vi "Update Wall State.vi"(10 "wall state in":T1, 11 "map in":refnum<data-value>) -> (2 "wall state out":T1, 3 "map out":refnum<data-value>)   [LabVIEW 2020, in "Great Wall.lvclass"]
uses:
  Great Wall.lvclass
  DS Square Library/Mapping/Map.ctl
  DS Square Library/Mapping/Square Status.ctl
  DS Square Library/Mapping/Square State.ctl
  DS Square Library/Mapping/Center of Mass.ctl
  Wall State.ctl
  Wall State Enum.ctl
  Type Defs/Direction Enum.ctl
  Common/Position.ctl
  SubVIs/Read-Only Globals.vi
  SubVIs/Globals (private).vi
  DS Square Library/DS Square.lvlib
  Common/Common.lvlib
  Square/Square.lvclass
  Type Defs/SB Type Defs.lvlib
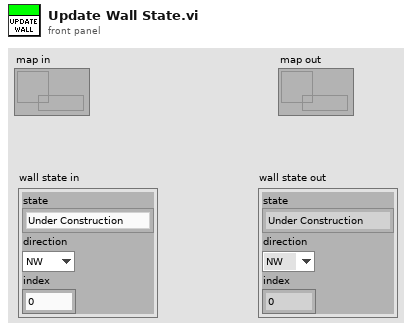
[diagram p1: front panel]
types:
  T1 = typedef "Great Wall.lvclass/Wall State.ctl" = cluster{"state":T2, "direction":T3, "index":i32}
  T2 = typedef "Great Wall.lvclass/Wall State Enum.ctl" = enum16{"Under Construction", "Hold", "Advance 1", "Advance 2", "Retreat"}
  T3 = typedef "SB Type Defs.lvlib/Direction Enum.ctl" = enum16{"NW", "N", "NE", "E", "SE", "S", "SW", "W"}
  T4 = typedef "DS Square.lvlib/Square State.ctl" = enum16{"Unknown", "Empty", "Occupied - Active", "Occupied - Cool Down", "Attacked", "Enemy", "Enemy Wall"}
  T5 = typedef "Common.lvlib/Position.ctl" = cluster{"Column":i32, "Row":i32}
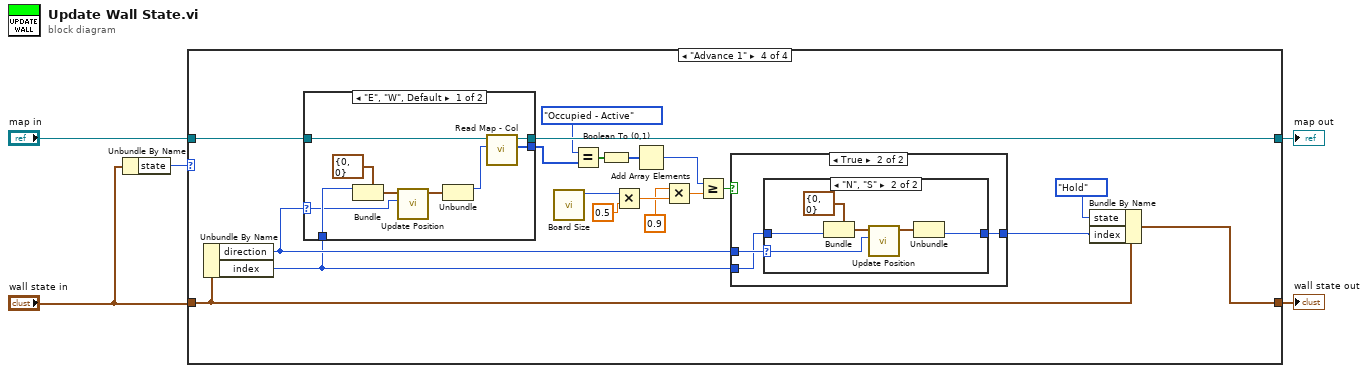
[diagram p0: block diagram]
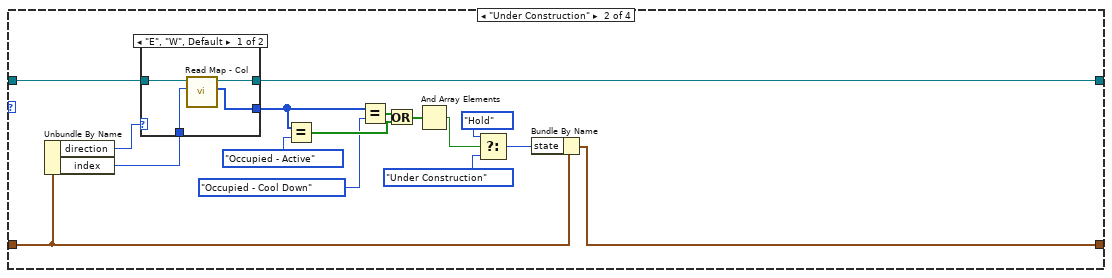
[diagram p3: hidden frame]
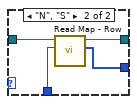
[diagram p4: hidden frame]
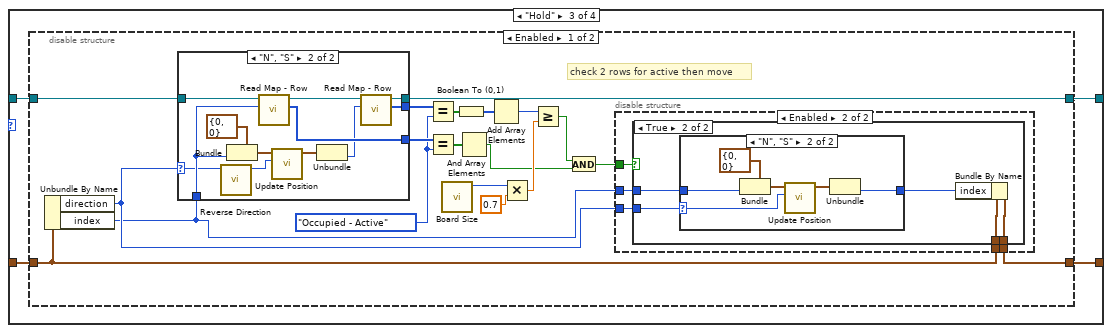
[diagram p5: hidden frame]
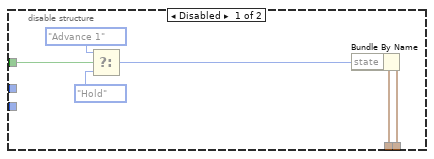
[diagram p6: hidden frame]
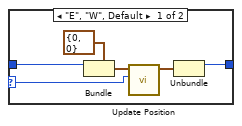
[diagram p8: hidden frame]
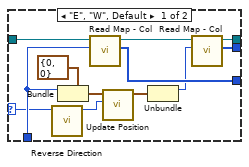
[diagram p9: hidden frame]
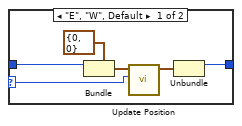
[diagram p12: hidden frame]
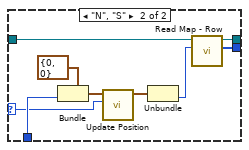
[diagram p13: hidden frame]
diagram:
  n1 = Unbundle By Name("wall state in") -> ("state"=w3:T2)
  n2 = case shown="\"Advance 1\"" w3 {
    tunnel: "map in" -> [w7 w17 w35 w127]
    tunnel: [w7 w16 w34 w126] -> w4
    tunnel: "wall state in" -> [w6 w13 w33 w125]
    tunnel: [w6 w8 w32 w128] -> w1
    frame Default {
    }
    frame "Under Construction" {
      n3 = Unbundle By Name(w13) -> ("direction"=w15:T3, "index"=w14:i32)
      n4 = case shown="\"E\", \"W\", Default" w15 {
        tunnel: w17 -> [w27 w31]
        tunnel: w14 -> [w24 w30]
        tunnel: [w26 w29] -> w16
        tunnel: [w25 w28] -> w19
        frame "E", "W", Default {
          n5 = call "Read Map - Col.vi"("Column"=w24, "map in"=w27) -> ("square states"=w25:T4[], "map out"=w26:refnum<data-value>)  [unwired: 8 in]
        }
        frame "N", "S" {
          n6 = call "Read Map - Row.vi"("Row"=w30, "map"=w31) -> ("square states"=w28:T4[], "map"=w29:refnum<data-value>)  [unwired: 8 in]
        }
      }
      n7 = Equal?(x=w19, y=Square_State."Occupied - Active" ("square state")) -> (x = y?=w22:bool[])
      n8 = Equal?(x=w19, y=Square_State."Occupied - Cool Down" ("square state")) -> (x = y?=w21:bool[])
      n9 = Or(x=w21, y=w22) -> (x .or. y?=w23:bool[])
      n10 = And Array Elements(Boolean array=w23) -> (logical AND=w12:bool)
      n11 = Select(t=Wall_State_Enum."Hold" ("state"), s=w12, f=Wall_State_Enum."Under Construction" ("state")) -> (s? t:f=w9:T2)
      n12 = Bundle By Name(cluster=w13, "state"=w9) -> (w8:T1)
    }
    frame "Hold" {
      n13 = disable-structure shown="Enabled" {
        disable-tunnel: w35 -> [w53 w109]
        disable-tunnel: [w52 w109] -> w34
        disable-tunnel: w33 -> [w51 w108]
        disable-tunnel: [w50 w108] -> w32
        frame Enabled {
          w47 = Square_State."Occupied - Active" ("square state")
          # "check 2 rows for active then move"
          n14 = Unbundle By Name(w51) -> ("direction"=w37:T3, "index"=w36:i32)
          n15 = case shown="\"N\", \"S\"" w37 {
            selector: w37 -> [w85 w97]
            tunnel: w53 -> [w95 w107]
            tunnel: w36 -> [w87 w99]
            tunnel: [w90 w102] -> w52
            tunnel: [w89 w101] -> w54
            tunnel: [w88 w100] -> w48
            frame "E", "W", Default {
              n16 = call "Reverse Direction.vi"("Direction in"=w85) -> ("Reverse Direction"=w84:i32)  [unwired: 10 in]
              n17 = Bundle(cluster=T5 {"Column"=0, "Row"=0} ("Position in"), "Column"=w87) -> (w93:T5)  [unwired: 1 in]
              n18 = call "Read Map - Col.vi"("Column"=w87, "map in"=w95) -> ("square states"=w89:T4[], "map out"=w91:refnum<data-value>)  [unwired: 8 in]
              n19 = call "Update Position.vi"("Direction"=w84, "Position in"=w93) -> ("Position out"=w92:T5)  [unwired: 9 in]
              n20 = Unbundle(w92) -> ("Column"=w86:i32)  [unwired: 1 out]
              n21 = call "Read Map - Col.vi"("Column"=w86, "map in"=w91) -> ("square states"=w88:T4[], "map out"=w90:refnum<data-value>)  [unwired: 8 in]
            }
            frame "N", "S" {
              n22 = call "Reverse Direction.vi"("Direction in"=w97) -> ("Reverse Direction"=w96:i32)  [unwired: 10 in]
              n23 = Bundle(cluster=T5 {"Column"=0, "Row"=0} ("Position in"), "Row"=w99) -> (w105:T5)  [unwired: 1 in]
              n24 = call "Read Map - Row.vi"("Row"=w99, "map"=w107) -> ("square states"=w101:T4[], "map"=w103:refnum<data-value>)  [unwired: 8 in]
              n25 = call "Update Position.vi"("Direction"=w96, "Position in"=w105) -> ("Position out"=w104:T5)  [unwired: 9 in]
              n26 = Unbundle(w104) -> ("Row"=w98:i32)  [unwired: 1 out]
              n27 = call "Read Map - Row.vi"("Row"=w98, "map"=w103) -> ("square states"=w100:T4[], "map"=w102:refnum<data-value>)  [unwired: 8 in]
            }
          }
          n28 = Equal?(x=w48, y=w47) -> (x = y?=w46:bool[])
          n29 = Equal?(x=w54, y=w47) -> (x = y?=w49:bool[])
          n30 = call "Board Size.vi"() -> ("Board Size"=w44:i32)  [unwired: 11 in]
          n31 = Boolean To (0,1)(Boolean=w46) -> (0, 1=w45:i16[])
          n32 = And Array Elements(Boolean array=w49) -> (logical AND=w39:bool)
          n33 = Add Array Elements(numeric array=w45) -> (sum=w42:i16)
          n34 = Multiply(x=w44, y=0.7) -> (x*y=w41:dbl)
          n35 = Greater Or Equal?(x=w42, y=w41) -> (x >= y?=w40:bool)
          n36 = And(x=w40, y=w39) -> (x .and. y?=w38:bool)
          n37 = disable-structure shown="Enabled" {
            disable-tunnel: w51 -> [w60 w61]
            disable-tunnel: [w56 w62] -> w50
            disable-tunnel: w38 -> [w55 w64]
            disable-tunnel: w37 -> [_ w65]
            disable-tunnel: w36 -> [_ w63]
            frame Disabled {
              n38 = Select(t=Wall_State_Enum."Advance 1" ("state"), s=w55, f=Wall_State_Enum."Hold" ("state")) -> (s? t:f=w57:T2)
              n39 = Bundle By Name(cluster=w60, "state"=w57) -> (w56:T1)
            }
            frame Enabled {
              n40 = case shown="True" w64 {
                tunnel: w65 -> [_ w71]
                tunnel: w63 -> [_ w70]
                tunnel: [w66 w69] -> w62
                tunnel: w61 -> [w66 w68]
                frame False {
                }
                frame True {
                  n41 = case shown="\"N\", \"S\"" w71 {
                    selector: w71 -> [w72 w78]
                    tunnel: w70 -> [w74 w80]
                    tunnel: [w73 w79] -> w67
                    frame "E", "W", Default {
                      n42 = Bundle(cluster=T5 {"Column"=0, "Row"=0} ("Position in"), "Column"=w74) -> (w76:T5)  [unwired: 1 in]
                      n43 = call "Update Position.vi"("Direction"=w72, "Position in"=w76) -> ("Position out"=w77:T5)  [unwired: 9 in]
                      n44 = Unbundle(w77) -> ("Column"=w73:i32)  [unwired: 1 out]
                    }
                    frame "N", "S" {
                      n45 = Bundle(cluster=T5 {"Column"=0, "Row"=0} ("Position in"), "Row"=w80) -> (w82:T5)  [unwired: 1 in]
                      n46 = call "Update Position.vi"("Direction"=w78, "Position in"=w82) -> ("Position out"=w83:T5)  [unwired: 9 in]
                      n47 = Unbundle(w83) -> ("Row"=w79:i32)  [unwired: 1 out]
                    }
                  }
                  n48 = Bundle By Name(cluster=w68, "index"=w67) -> (w69:T1)
                }
              }
            }
          }
        }
        frame Disabled {
        }
      }
    }
    frame "Advance 1" {
      n49 = Unbundle By Name(w125) -> ("direction"=w120:T3, "index"=w119:i32)
      n50 = case shown="\"E\", \"W\", Default" w120 {
        selector: w120 -> [w145 w154]
        tunnel: w127 -> [w153 w162]
        tunnel: w119 -> [w147 w156]
        tunnel: [w149 w158] -> w126
        tunnel: [w148 w157] -> w122
        frame "E", "W", Default {
          n51 = Bundle(cluster=T5 {"Column"=0, "Row"=0} ("Position in"), "Column"=w147) -> (w151:T5)  [unwired: 1 in]
          n52 = call "Update Position.vi"("Direction"=w145, "Position in"=w151) -> ("Position out"=w150:T5)  [unwired: 9 in]
          n53 = Unbundle(w150) -> ("Column"=w146:i32)  [unwired: 1 out]
          n54 = call "Read Map - Col.vi"("Column"=w146, "map in"=w153) -> ("square states"=w148:T4[], "map out"=w149:refnum<data-value>)  [unwired: 8 in]
        }
        frame "N", "S" {
          n55 = Bundle(cluster=T5 {"Column"=0, "Row"=0} ("Position in"), "Row"=w156) -> (w160:T5)  [unwired: 1 in]
          n56 = call "Update Position.vi"("Direction"=w154, "Position in"=w160) -> ("Position out"=w159:T5)  [unwired: 9 in]
          n57 = Unbundle(w159) -> ("Row"=w155:i32)  [unwired: 1 out]
          n58 = call "Read Map - Row.vi"("Row"=w155, "map"=w162) -> ("square states"=w157:T4[], "map"=w158:refnum<data-value>)  [unwired: 8 in]
        }
      }
      n59 = call "Board Size.vi"() -> ("Board Size"=w117:i32)  [unwired: 11 in]
      n60 = Equal?(x=Square_State."Occupied - Active" ("square state"), y=w122) -> (x = y?=w123:bool[])
      n61 = Boolean To (0,1)(Boolean=w123) -> (0, 1=w124:i16[])
      n62 = Multiply(x=w117, y=0.5) -> (x*y=w116:dbl)
      n63 = Add Array Elements(numeric array=w124) -> (sum=w113:i16)
      n64 = Multiply(x=0.9, y=w116) -> (x*y=w114:dbl)
      n65 = Greater Or Equal?(x=w113, y=w114) -> (x >= y?=w110:bool)
      n66 = case shown="True" w110 {
        tunnel: w120 -> [_ w132]
        tunnel: w119 -> [w129 w131]
        tunnel: [w129 w130] -> w111
        frame False {
        }
        frame True {
          n67 = case shown="\"N\", \"S\"" w132 {
            selector: w132 -> [w133 w139]
            tunnel: w131 -> [w135 w141]
            tunnel: [w134 w140] -> w130
            frame "E", "W", Default {
              n68 = Bundle(cluster=T5 {"Column"=0, "Row"=0} ("Position in"), "Column"=w135) -> (w137:T5)  [unwired: 1 in]
              n69 = call "Update Position.vi"("Direction"=w133, "Position in"=w137) -> ("Position out"=w138:T5)  [unwired: 9 in]
              n70 = Unbundle(w138) -> ("Column"=w134:i32)  [unwired: 1 out]
            }
            frame "N", "S" {
              n71 = Bundle(cluster=T5 {"Column"=0, "Row"=0} ("Position in"), "Row"=w141) -> (w143:T5)  [unwired: 1 in]
              n72 = call "Update Position.vi"("Direction"=w139, "Position in"=w143) -> ("Position out"=w144:T5)  [unwired: 9 in]
              n73 = Unbundle(w144) -> ("Row"=w140:i32)  [unwired: 1 out]
            }
          }
        }
      }
      n74 = Bundle By Name(cluster=w125, "state"=Wall_State_Enum."Hold", "index"=w111) -> (w128:T1)
    }
  }
  "map out" <- w4
  "wall state out" <- w1
